vi "Test WARNING-Logger.vi"(8 "error in":errorcluster) -> (0 "error out":errorcluster)   [LabVIEW 2016, in "UT_Helper.lvlib"]
doc: "Test correct function of the Warning-Logger."
uses:
  UT_Helper.lvlib
  Source/HSE-Logger/LogLevel.ctl
  Source/HSE-Logger/LogRecord/LogRecord.lvclass/LogRecord.ctl
  Source/HSE-Logger/Handler/UserEventHandler/UserEventHandler.lvclass
  C:/Users/admin/_Git/hse-logger/Source/HSE-Logger/Handler/Handler.lvclass
  <vilib>/addons/_JKI Toolkits/Caraya/classes/Test/Test.lvclass
  Source/HSE-Logger/hse-logger.lvlib
  Source/HSE-Logger/LogRecord/LogRecord.lvclass
  <vilib>/addons/_JKI Toolkits/Caraya/classes/Assert/Assert.lvclass
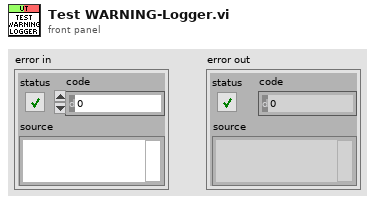
[diagram p1: front panel]
types:
  T1 = typedef "hse-logger.lvlib/LogLevel.ctl" = enum16{"DEBUG", "INFO", "WARNING", "ERROR", "CRITICAL"}
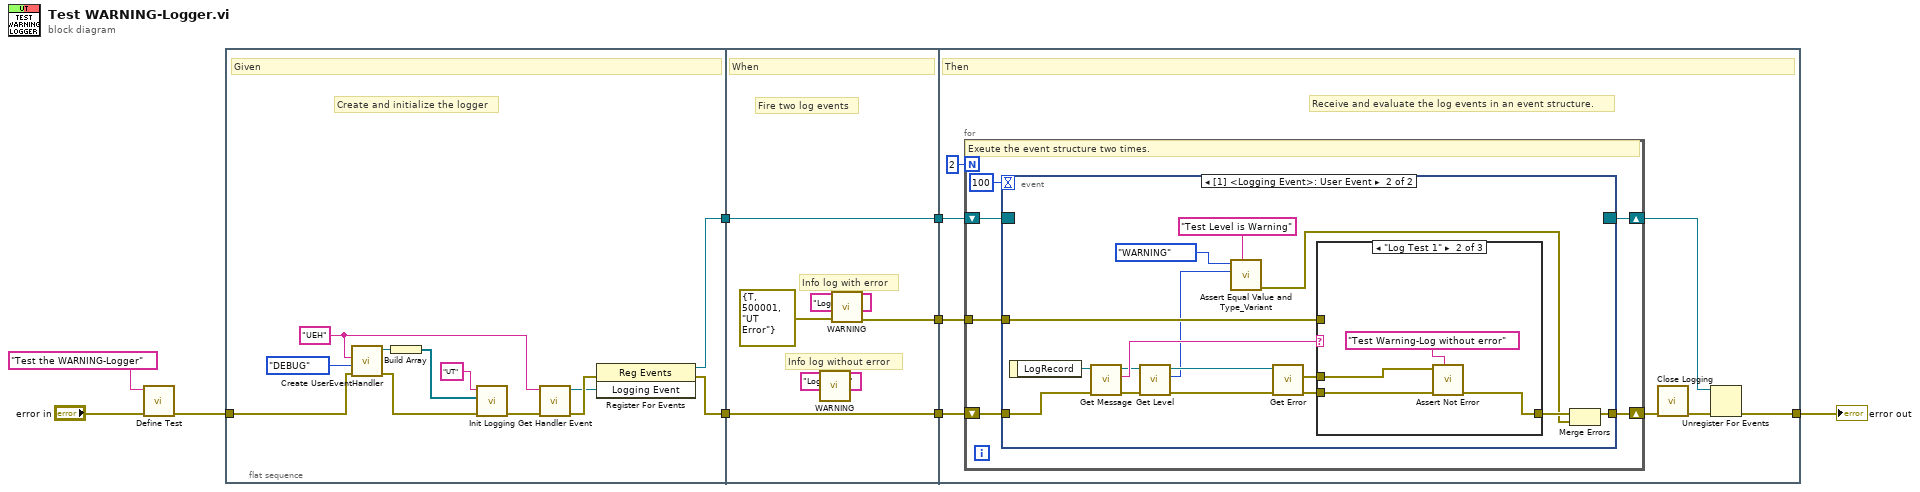
[diagram p0: block diagram]
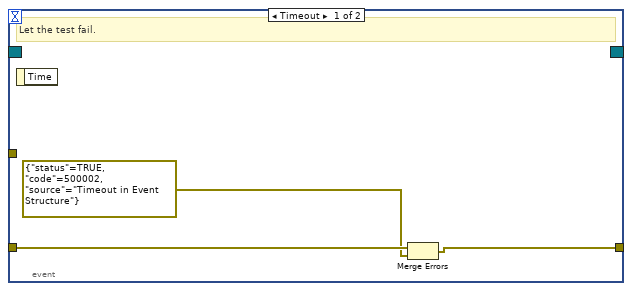
[diagram p2: hidden frame]
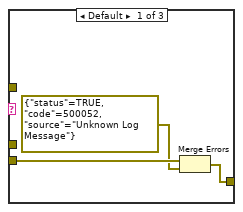
[diagram p3: hidden frame]
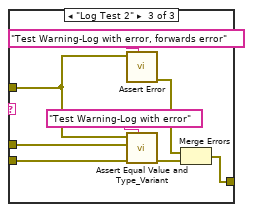
[diagram p4: hidden frame]
diagram:
  n1 = call <vilib>:"Define Test.vi"("error in (no error)"="error in", "Label (VI Title)"="Test the WARNING-Logger") -> ("error out"=w6:errorcluster)  [unwired: 8 in, 1 out]
  n2 = flat-sequence {
    tunnel: w6 -> [w20]
    tunnel: [w17] -> w9
    tunnel: [w12] -> w2
    tunnel: w9 -> [w27]
    tunnel: [w27] -> w5
    tunnel: w2 -> [w23]
    tunnel: [w23] -> w1
    tunnel: [w25] -> w4
    tunnel: [w31] -> w8
    tunnel: w5 -> [w35]
    tunnel: w1 -> [w30]
    tunnel: w4 -> [w34]
    frame #0 {
      w11 = "UEH" ("Name")
      # "Create and initialize the logger"
      # "Given"
      n3 = call "Create UserEventHandler.vi"("error in"=w20, "Level"=LogLevel."DEBUG", "Name"=w11) -> ("error out"=w19:errorcluster, "UserEventHandler out"=w16:refnum<class "UserEventHandler.lvclass">)  [unwired: 7 in]
      n4 = Build Array(w16) -> (w15:refnum<class "UserEventHandler.lvclass">[])
      n5 = call "Init Logging.vi"("error in"=w19, "Handlers"=w15, "Name"="UT") -> ("error out"=w18:errorcluster)  [unwired: 8 in]
      n6 = call "Get Handler Event.vi"("error in"=w18, "Name"=w11) -> ("error out"=w21:errorcluster, "Logging Event"=w13:refnum<user-event>)  [unwired: 8 in]
      n7 = register-events(error in=w21, w13) -> (reference out=w12:refnum<event-registration>, error out=w17:errorcluster)  [unwired: 1 in]
    }
    frame #1 {
      # "Info log with error"
      # "Info log without error"
      # "Fire two log events"
      # "When"
      n8 = call "WARNING.vi"("Message"="Log Test 1") -> ()  [unwired: 10 in, 1 out]
      n9 = call "WARNING.vi"("Message"="Log Test 2", "error in"=errorcluster {"status"=TRUE, "code"=500001, "source"="UT Error"}) -> ("error out"=w25:errorcluster)  [unwired: 9 in]
    }
    frame #2 {
      # "Receive and evaluate the log events in an event structure."
      # "Then"
      n10 = for {
        N: 2 -> [_]
        shift-right: [w40] -> w33
        shift-left: w35 -> [w41]
        tunnel: w34 -> [w39]
        shift-right: [w36] -> w28
        shift-left: w30 -> [w38]
        # "Exeute the event structure two times."
        n11 = event shown="[1] <Logging Event>: User Event" {
          selector: w38 -> [_ _]
          dyn-events: [_ _] -> w36
          timeout: 100 -> [_ _]
          tunnel: w41 -> [w44 w60]
          tunnel: [w42 w53] -> w40
          tunnel: w39 -> [_ w56]
          event Timeout {
            # "Let the test fail."
            n12 = event-data() -> ()  [unwired: 1 in, 1 out]
            n13 = Merge Errors(w44, errorcluster {"status"=TRUE, "code"=500002, "source"="Timeout in Event Structure"} ("error out")) -> (w42:errorcluster)
          }
          event User Event {
            n14 = event-data() -> ("LogRecord"=w51:refnum<class "LogRecord.lvclass">)  [unwired: 1 in]
            n15 = call "Get Message.vi"("error in"=w60, "LogRecord in"=w51) -> ("error out"=w55:errorcluster, "Message"=w50:string, "LogRecord out"=w49:refnum<class "LogRecord.lvclass">)  [unwired: 7 in]
            n16 = call "Get Level.vi"("error in"=w55, "LogRecord in"=w49) -> ("error out"=w54:errorcluster, "Level"=w47:T1, "LogRecord out"=w48:refnum<class "LogRecord.lvclass">)  [unwired: 7 in]
            n17 = call <vilib>:"Assert Equal Value and Type_Variant.vi"("Label"="Test Level is Warning", "Y"=w47, "X"=LogLevel."WARNING" ("Level")) -> ("error out"=w52:errorcluster)  [unwired: 7 in, 1 out]
            n18 = call "Get Error.vi"("error in"=w54, "LogRecord in"=w48) -> ("error out"=w58:errorcluster, "Error"=w59:errorcluster)  [unwired: 7 in, 1 out]
            n19 = case shown="\"Log Test 1\"" w50 {
              tunnel: w59 -> [_ w66 w73]
              tunnel: w58 -> [w63 w67 w75]
              tunnel: [w61 w65 w71] -> w57
              tunnel: w56 -> [_ _ w72]
              frame Default {
                n20 = Merge Errors(w63, errorcluster {"status"=TRUE, "code"=500052, "source"="Unknown Log Message"} ("error out")) -> (w61:errorcluster)
              }
              frame "Log Test 1" {
                n21 = call <vilib>:"Assert Not Error.vi"("Label"="Test Warning-Log without error", "error in (no error)"=w67, "Not Error?"=w66) -> ("error out"=w65:errorcluster)  [unwired: 7 in, 1 out]
              }
              frame "Log Test 2" {
                n22 = call <vilib>:"Assert Error.vi"("Label"="Test Warning-Log with error, forwards error", "Error?"=w72) -> ("error out"=w70:errorcluster)  [unwired: 8 in, 1 out]
                n23 = call <vilib>:"Assert Equal Value and Type_Variant.vi"("Label"="Test Warning-Log with error", "error in (no error)"=w75, "Y"=w73, "X"=w72) -> ("error out"=w74:errorcluster)  [unwired: 6 in, 1 out]
                n24 = Merge Errors(w70, w74) -> (w71:errorcluster)
              }
            }
            n25 = Merge Errors(w57, w52) -> (w53:errorcluster)
          }
        }
      }
      n26 = call "Close Logging.vi"("error in"=w33) -> ("error out"=w32:errorcluster)  [unwired: 10 in]
      n27 = Unregister For Events(event registration refnum=w28, error in=w32) -> (error out=w31:errorcluster)
    }
  }
  "error out" <- w8
